vi "AQT_get_board_info.vi"(11 "hnd":u32) -> (1 "Model Number":string, 2 "Board ID":string, 3 "hnd out":u32)   [LabVIEW 2013]
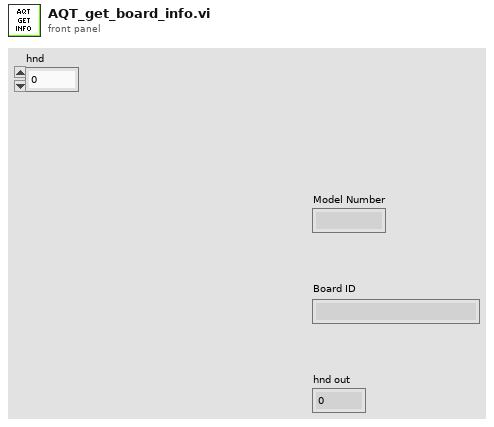
[diagram p1: front panel]
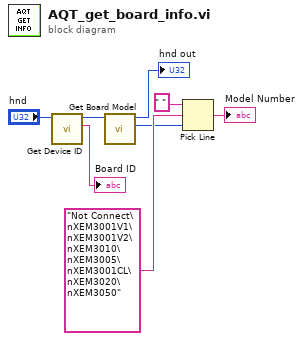
[diagram p0: block diagram]
diagram:
  n1 = call <userlib>:"Get Device ID.vi"("hnd"="hnd") -> ("buf out"=→"Board ID":string, "hnd out"=w2:u32)  [unwired: 9 in]
  n2 = call <userlib>:"Get Board Model.vi"("hnd"=w2) -> ("function return"=w4:u32, "hnd out"=→"hnd out":u32)  [unwired: 9 in]
  n3 = Pick Line(string ("")=" ", multi-line string="Not Connect\nXEM3001V1\nXEM3001V2\nXEM3010\nXEM3005\nXEM3001CL\nXEM3020\nXEM3050", line index=w4) -> (output string=→"Model Number":string)
